vi "트리거.vi"() -> ()   [LabVIEW 2018]
uses:
  <vilib>/DAQmx/create/channels.llb/DAQmx Create Channel (AI-Voltage-Basic).vi
  <vilib>/DAQmx/configure/timing.llb/DAQmx Timing (Sample Clock).vi
  <vilib>/DAQmx/read.llb/DAQmx Read (Analog Wfm 1Chan NSamp).vi
  <vilib>/DAQmx/configure/trigger.llb/DAQmx Start Trigger (Digital Edge).vi
panel:
  out "error out":errorcluster caption="에러 출력"
  in  "samples per channel":i32=1000 caption="채널당 샘플"
  in  "sample mode":i32(ring)=10178 caption="샘플 모드" items=["유한 샘플"=10178, "연속 샘플"=10123, "하드웨어 타이밍에 의한 단일 포인트"=12522]
  in  "rate":dbl=1000.0 caption="속도" format="%0.2f"
  out "data":waveform(dbl)(graph) caption="데이터"
  in  "number of samples per channel":i32=-1 caption="채널당 샘플 개수"
  in  "timeout":dbl=10.0 caption="타임아웃" format="%0.2f"
  in  "source":tag
  in  "edge":i32(ring)=10280 caption="에지" items=["상승"=10280, "하강"=10171]
  in  "channel name":string caption="할당된 이름"
  in  "minimum value":dbl=-5.0 caption="최소값" format="%0.2f"
  in  "input terminal configuration":i32(ring)=-1 caption="입력 터미널 설정" items=["기본"=-1, "RSE"=10083, "NRSE"=10078, "차동"=10106, "유사 차동"=12529]
  in  "maximum value":dbl=5.0 caption="최대값" format="%0.2f"
  in  "physical channels":tag caption="물리적 채널"
  in  "error in":errorcluster caption="에러 입력"
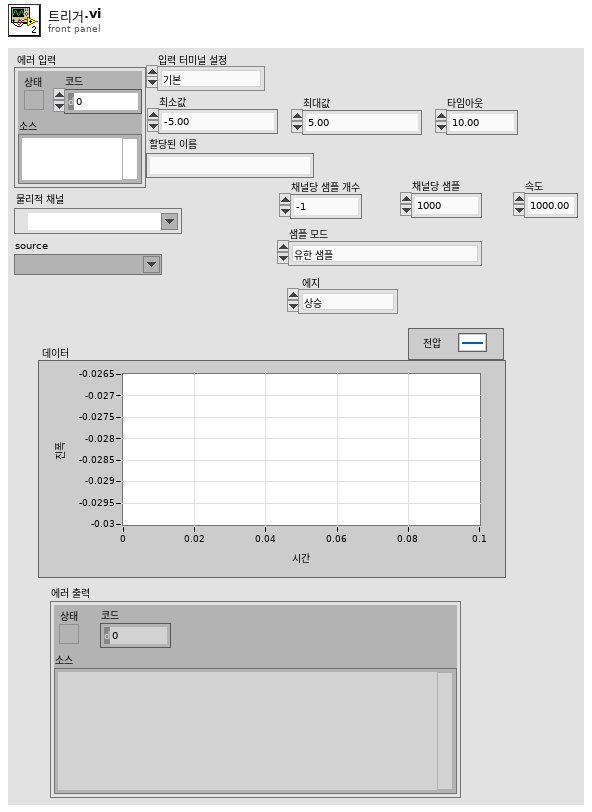
[diagram p1: front panel]
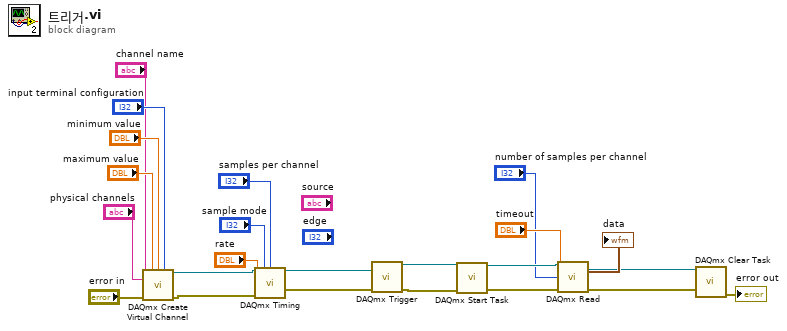
[diagram p0: block diagram]
diagram:
  n1 = call-poly <vilib>:"DAQmx Create Virtual Channel.vi"("maximum value"="maximum value", "minimum value"="minimum value", "input terminal configuration"="input terminal configuration", "physical channels"="physical channels", "name to assign"="channel name", "error in"="error in") -> ("task out"=w22:refnum<k21>, "error out"=w21:errorcluster)  [unwired: 8 in]
  n2 = call-poly <vilib>:"DAQmx Timing.vi"("task/channels in"=w22, "sample mode"="sample mode", "samples per channel"="samples per channel", "rate"="rate", "error in"=w21) -> ("task out"=w15:refnum<k21>, "error out"=w14:errorcluster)  [unwired: 9 in]
  n3 = call-poly <vilib>:"DAQmx Trigger.vi"("task/channels in"=w15, "error in"=w14) -> ("task out"=w13:refnum<k21>, "error out"=w12:errorcluster)  [unwired: 12 in]
  n4 = call <vilib>:"DAQmx Start Task.vi"("task/channels in"=w13, "error in"=w12) -> ("task out"=w11:refnum<k21>, "error out"=w10:errorcluster)  [unwired: 12 in]
  n5 = call-poly <vilib>:"DAQmx Read.vi"("task/channels in"=w11, "number of samples per channel"="number of samples per channel", "timeout"="timeout", "error in"=w10) -> ("task out"=w3:refnum<k21>, "data"=→"data":waveform(dbl), "error out"=w2:errorcluster)  [unwired: 9 in]
  n6 = call <vilib>:"DAQmx Clear Task.vi"("task in"=w3, "error in"=w2) -> ("error out"=→"error out":errorcluster)  [unwired: 13 in]
